vi "stop_loop.vi"() -> ()   [LabVIEW 2024]
panel:
  in  "Stop loop":bool
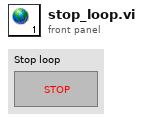
[diagram p1: front panel]
diagram:
